vi "MecaDrivePoseEst2_BufferDuration.vi"() -> (3 "Buffer Duration (Sec)":dbl)   [LabVIEW 2019, in "Trajectory_Library.lvlib"]
doc: "Gets the maximum duration for the Time Interp Variant buffer.\n\nThis is an internal routine. It should NOT be called by the end user."
uses:
  Trajectory_Library.lvlib
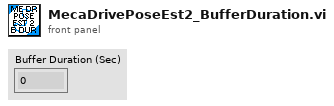
[diagram p1: front panel]
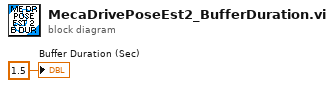
[diagram p0: block diagram]
diagram:
  "Buffer Duration (Sec)" <- 1.5 ("Buffer Duration (Sec)")
